vi "Latch Data.vi"(8 "error in (no error)":errorcluster, 10 "Time Stamp":timestamp=timestamp(3631881134.247515 s since 1904-01-01), 11 "dt":dbl=2000.0) -> (0 "error out":errorcluster, 3 "Waveform Array":waveform(dbl)[](array[waveform])=[{"t0"=timestamp(3631881134.247515 s since 1904-01-01), "dt"=2000.0, "Y"=[0.0], "attributes"=variant("NI_ChannelName"=variant(string "Pump 1 Flow"))}])   [LabVIEW 2018, in "Waveform Loop.lvlib"]
uses:
  Waveform Loop.lvlib
  Tag VIs/Tag FGV Operation Enum.ctl
  <vilib>/ptbypt/NI_PtbyPt.lvlib
  Shared Variables/Dynamic Shared Variables.lvlib
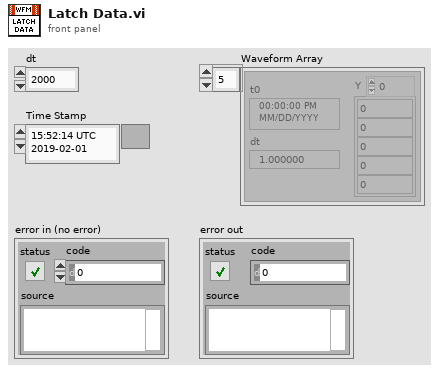
[diagram p1: front panel]
types:
  T1 = typedef "Tag FGV Operation Enum.ctl" = enum16{"Init", "Set Notification Queue", "Create Tag", "Commit", "Write Tag (Numeric)", "Write Tag (Boolean)", "Read All Tags", "Read One Tag", "Delete Tag Category", "Set Alarm Parameters (Numeric)", "Set Alarm Parameters (Boolean)", "Enable All Alarms", "Disable All Alarms", "Delete All Tags", "Read Alarms", "Ack Alarm"}
  T2 = enum32{"u32BitField", "bool", "double", "string", "int8", "uint8", "int16", "uint16", "int32", "uint32", "int64", "uint64", "single", "double waveform", "int16 waveform", "array of boolean", "array of int8", "array of uint8", "array of int16", "array of uint16", "array of int32", "array of uint32", "array of int64", "array of uint64", "array of single", "array of double", "array of double waveform", "array of int16 waveform", "array of string", "variant", "timestamp", "fixed point", "custom"}
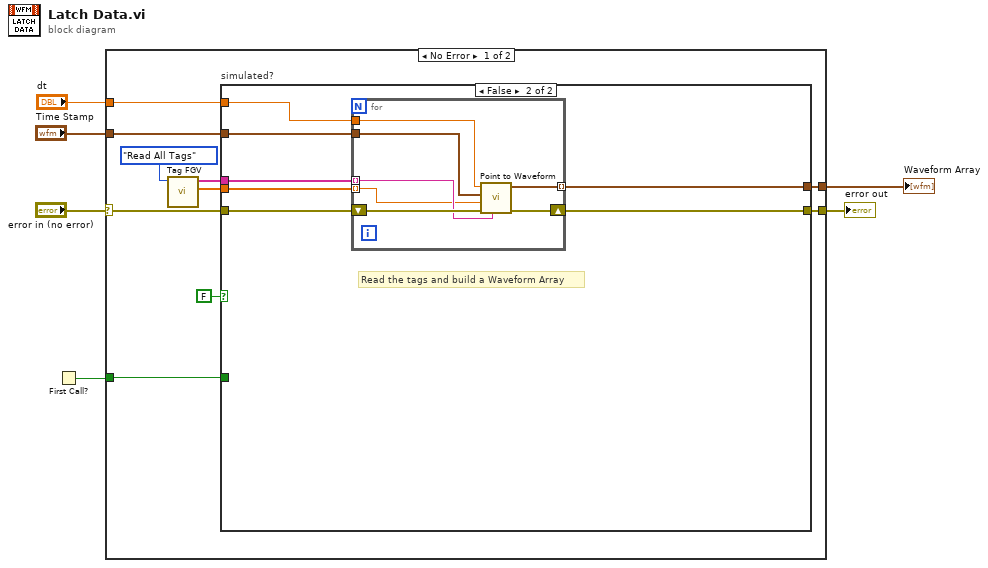
[diagram p0: block diagram]
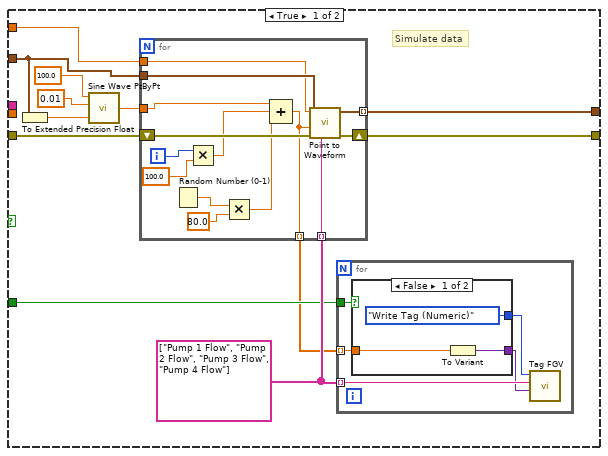
[diagram p2: hidden frame]
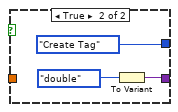
[diagram p3: hidden frame]
diagram:
  n1 = First Call?() -> (First Call?: T/F=w1:bool)
  n2 = case shown="No Error" "error in (no error)" {
    selector: "error in (no error)" -> [w15 w68]
    tunnel: [w12 _] -> w6
    tunnel: [w16 w68] -> w5
    tunnel: "dt" -> [w13 _]
    tunnel: "Time Stamp" -> [w14 _]
    tunnel: w1 -> [w7 _]
    frame No Error {
      n3 = call "Tag FGV.vi"("Operation"=Tag_FGV_Operation_Enum."Read All Tags") -> ("Tag Values"=w8:dbl[], "Tag Names"=w9:string[])  [unwired: 5 in, 4 out]
      n4 = case "simulated?" shown="False" FALSE {
        tunnel: [w28 w60] -> w16
        tunnel: w15 -> [w27 w59]
        tunnel: w14 -> [w23 w58]
        tunnel: w13 -> [w22 w57]
        tunnel: [w21 w56] -> w12
        tunnel: w9 -> [_ w55]
        tunnel: w8 -> [_ w54]
        tunnel: w7 -> [w18 _]
        frame True {
          w19 = string[] ["Pump 1 Flow", "Pump 2 Flow", "Pump 3 Flow", "Pump 4 Flow"]
          # "Simulate data"
          n5 = To Extended Precision Float(1:w23) -> (0:w24:ext)
          n6 = call <vilib>:"Sine Wave PtByPt.vi"("time"=w24, "frequency"=0.01, "amplitude"=100.0) -> ("sine wave"=w20:dbl)  [unwired: 1 in]
          n7 = for {
            tunnel: [w53] -> w21 mode=indexing
            tunnel: w19 -> [w51] mode=indexing
            tunnel: w23 -> [w49]
            tunnel: w22 -> [w48]
            shift-right: [w52] -> w28
            shift-left: w27 -> [w50]
            tunnel: w20 -> [w46]
            tunnel: [w40] -> w17 mode=indexing
            i -> [w44]
            n8 = Random Number (0-1)() -> (number: 0 to 1=w47:dbl)
            n9 = Multiply(x=w44, y=100.0 ("value")) -> (x*y=w42:dbl)
            n10 = Multiply(x=w47, y=80.0) -> (x*y=w41:dbl)
            n11 = Compound Arithmetic op=ADD(w46, w42, w41) -> (w40:dbl)
            n12 = call "Point to Waveform.vi"("Channel name"=w51, "error in (no error)"=w50, "data"=w40, "Time Stamp"=w49, "dt"=w48) -> ("error out"=w52:errorcluster, "Waveform"=w53:waveform(dbl))  [unwired: 5 in]
          }
          n13 = for {
            tunnel: w19 -> [w33] mode=indexing
            tunnel: w18 -> [w32]
            tunnel: w17 -> [w29] mode=indexing
            n14 = case shown="False" w32 {
              tunnel: [Tag_FGV_Operation_Enum."Write Tag (Numeric)" ("Operation") Tag_FGV_Operation_Enum."Create Tag" ("Operation")] -> w31
              tunnel: [w34 w38] -> w30
              tunnel: w29 -> [w35 _]
              frame False {
                n15 = To Variant(anything=w35) -> (Variant=w34:variant)
              }
              frame True {
                n16 = To Variant(anything=T2."double" ("data type")) -> (Variant=w38:variant)
              }
            }
            n17 = call "Tag FGV.vi"("Data"=w30, "Tag Name"=w33, "Operation"=w31) -> ()  [unwired: 3 in, 6 out]
          }
        }
        frame False {
          # "Read the tags and build a Waveform Array"
          n18 = for {
            tunnel: [w67] -> w56 mode=indexing
            tunnel: w58 -> [w64]
            tunnel: w57 -> [w63]
            shift-right: [w66] -> w60
            shift-left: w59 -> [w65]
            tunnel: w55 -> [w62] mode=indexing
            tunnel: w54 -> [w61] mode=indexing
            n19 = call "Point to Waveform.vi"("Channel name"=w62, "error in (no error)"=w65, "data"=w61, "Time Stamp"=w64, "dt"=w63) -> ("error out"=w66:errorcluster, "Waveform"=w67:waveform(dbl))  [unwired: 5 in]
          }
        }
      }
    }
    frame Error {
    }
  }
  "Waveform Array" <- w6
  "error out" <- w5
